vi "Baum Welch Algorithm.vi"(9 "#iterations":i32=100, 10 "Observed states":i32[](array[numeric]), 11 "Init HMM":T1) -> (0 "Pre Estimated HMM":T1, 1 "#iterations":i32, 2 "Probability":dbl[](array[numeric]), 3 "Estimated HMM":T1)   [LabVIEW 2014, in "HMM.lvlib"]
uses:
  HMM.lvlib
  Control/HMM Cluster.ctl
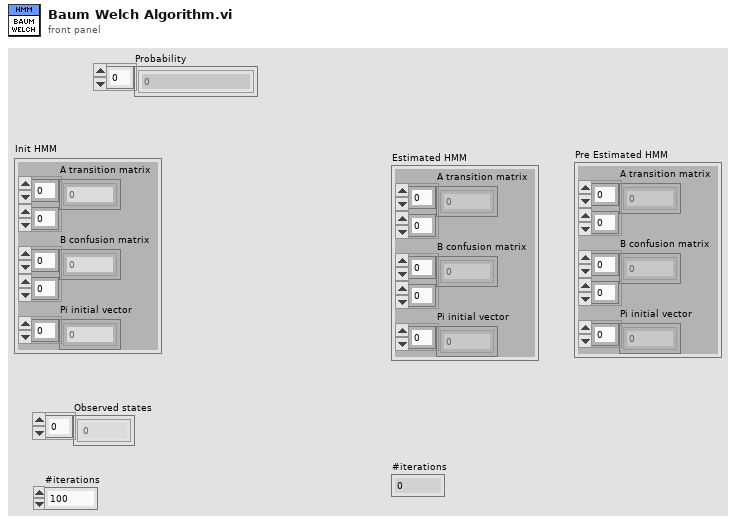
[diagram p1: front panel]
types:
  T1 = typedef "HMM.lvlib/HMM Cluster.ctl" = cluster{"A transition matrix":dbl[][], "B confusion matrix":dbl[][], "Pi initial vector":dbl[]}
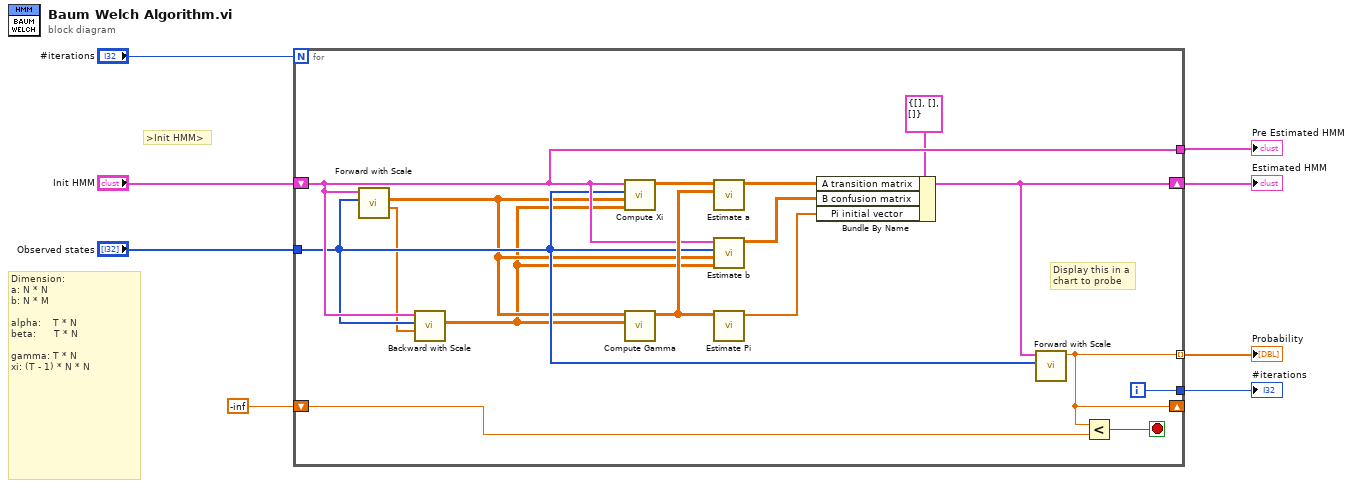
[diagram p0: block diagram]
diagram:
  # ">Init HMM>"
  # "Dimension:\na: N * N\nb: N * M\n\nalpha:    T * N\nbeta:      T * N\n\ngamma: T * N\nxi: (T - 1) * N * N"
  n1 = for {
    N: "#iterations" -> [_]
    tunnel: "Observed states" -> [w14]
    shift-right: [w15] -> w1
    shift-left: "Init HMM" -> [w16]
    tunnel: [w13] -> w6 mode=indexing
    shift-right: [w13] -> _
    shift-left: -inf ("Probability") -> [w19]
    tunnel: [w17] -> w4
    tunnel: [w16] -> w2
    i -> [w17]
    stop <- w18 stop-if-true
    # "Display this in a\nchart to probe"
    n2 = call "Forward with Scale.vi"("O Observed Sequence"=w14, "HMM Cluster"=w16) -> ("Scale factor"=w12:dbl[], "Scaled Alpha"=w11:dbl[][])  [unwired: 6 in, 2 out]
    n3 = call "Backward with Scale.vi"("Scale factor"=w12, "O Observed Sequence"=w14, "HMM Cluster"=w16) -> ("Beta Partial Probalility"=w10:dbl[][])  [unwired: 8 in]
    n4 = call "Compute Xi.vi"("Beta"=w10, "Alpha"=w11, "Observed sequence O"=w14, "HMM Cluster"=w16) -> ("Xi"=w24:dbl[][][])  [unwired: 7 in]
    n5 = call "Compute Gamma.vi"("Beta"=w10, "Alpha"=w11) -> ("Gamma"=w22:dbl[][])  [unwired: 9 in]
    n6 = call "Estimate a.vi"("Gamma"=w22, "Xi"=w24) -> ("Estimated a"=w20:dbl[][])  [unwired: 9 in]
    n7 = call "Estimate b.vi"("Beta"=w10, "Alpha"=w11, "Observed states"=w14, "HMM Cluster"=w16) -> ("Estimated b"=w21:dbl[][])  [unwired: 7 in]
    n8 = call "Estimate Pi.vi"("Gamma"=w22) -> ("Estimated Pi"=w23:dbl[])  [unwired: 10 in]
    n9 = Bundle By Name(cluster=T1 {"A transition matrix"=[], "B confusion matrix"=[], "Pi initial vector"=[]} ("HMM Cluster"), "A transition matrix"=w20, "B confusion matrix"=w21, "Pi initial vector"=w23) -> (w15:T1)
    n10 = call "Forward with Scale.vi"("O Observed Sequence"=w14, "HMM Cluster"=w15) -> ("Log10(Prob)"=w13:dbl)  [unwired: 6 in, 3 out]
    n11 = Less?(x=w13, y=w19) -> (x < y?=w18:bool)
  }
  "Estimated HMM" <- w1
  "Probability" <- w6
  "#iterations" <- w4
  "Pre Estimated HMM" <- w2
